vi "Update_display.vi"(8 "error in (no error)":errorcluster, 9 "Display":string, 11 "Display_Console_UI in":refnum<class "Display_Console_UI.lvclass">) -> (0 "error out":errorcluster, 3 "Display_Console_UI out":refnum<class "Display_Console_UI.lvclass">)   [LabVIEW 2025, in "Display_Console_UI.lvlib" / "Display_Console_UI.lvclass"]
uses:
  Display_Console_UI.lvclass
  Display_Console_UI.lvclass/Display_Console_UI.ctl
  <vilib>/event_ctls.llb/usereventprio.ctl
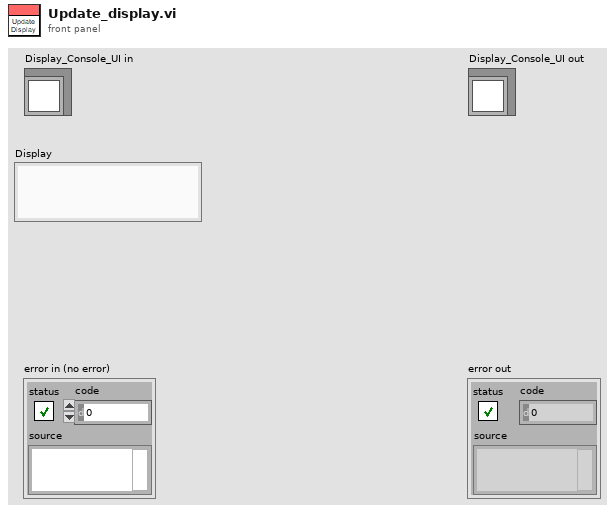
[diagram p1: front panel]
types:
  T1 = typedef "usereventprio.ctl" = enum32{"high priority", "normal priority"}
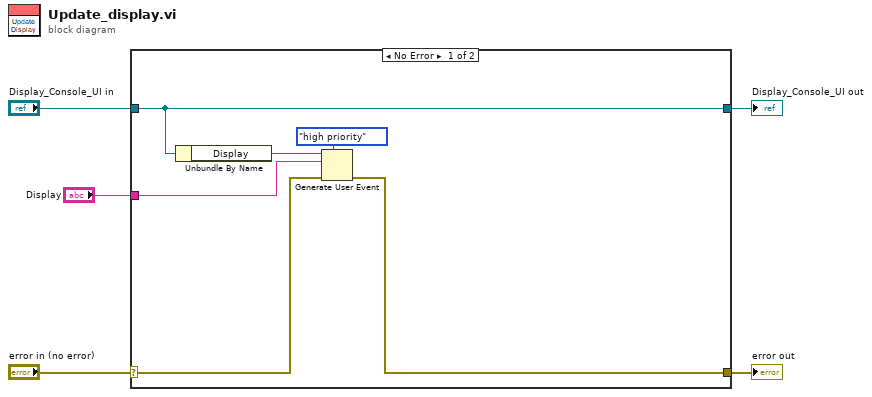
[diagram p0: block diagram]
diagram:
  n1 = case shown="No Error" "error in (no error)" {
    selector: "error in (no error)" -> [w7 w13]
    tunnel: [w6 w13] -> w4
    tunnel: [w11 w12] -> w2
    tunnel: "Display_Console_UI in" -> [w11 w12]
    tunnel: "Display" -> [w8 _]
    frame No Error {
      n2 = Unbundle By Name(w11) -> ("Display"=w10:refnum<user-event>)
      n3 = Generate User Event(priority (normal)=usereventprio."high priority", user event=w10, event data cluster=w8, error in=w7) -> (error out=w6:errorcluster)  [unwired: 1 out]
    }
    frame Error {
    }
  }
  "error out" <- w4
  "Display_Console_UI out" <- w2
